vi "New.vi"(8 "Error In":errorcluster) -> (0 "Error Out":errorcluster, 3 "Compiler":refnum<class "Compiler.lvclass">)   [LabVIEW 2018, in "Toolkit.lvlib" / "Compiler.lvclass"]
uses:
  Compiler.lvclass
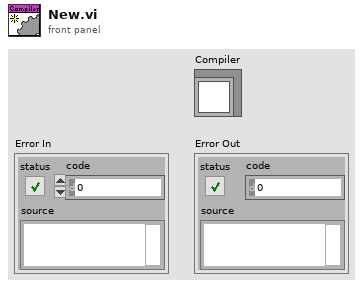
[diagram p1: front panel]
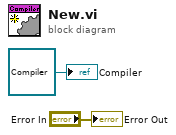
[diagram p0: block diagram]
diagram:
  "Compiler" <- refnum<class "Compiler.lvclass"> refnum ("Toolkit.lvlib:Compiler.lvclass")
  "Error Out" <- "Error In"
